vi "Stop Listener.vi"(8 "error in (no error)":errorcluster, 11 "Server Controller in":refnum<class "Server Controller.lvclass">) -> (0 "error out":errorcluster, 3 "Server Controller out":refnum<class "Server Controller.lvclass">)   [LabVIEW 2026, in "Server Controller.lvlib" / "Server Controller.lvclass"]
uses:
  Server Controller.lvclass
  <vilib>/ActorFramework/Message Enqueuer/Message Enqueuer.lvclass
  Server Controller.lvclass/Server Controller.ctl
  <vilib>/ActorFramework/Message Enqueuer/Message Enqueuer.lvclass/Message Enqueuer.ctl
  <vilib>/ActorFramework/Message Enqueuer/Enqueue.vi
  <vilib>/ActorFramework/Stop Msg/Stop Msg.lvclass
  C:/Program Files/National Instruments/LabVIEW 2026/vi.lib/ActorFramework/Message/Message.lvclass
  <vilib>/ActorFramework/Message Priority Queue/Priority Enqueue.vi
  recovery/packages/ni_lib_linked_network_actor-1.2.0.19-9492AF5A82/File Group 0/vi.lib/NI/Actors/Linked Network Actor/Linked Network Actor Messages/Disconnect Msg/Disconnect Msg.lvclass
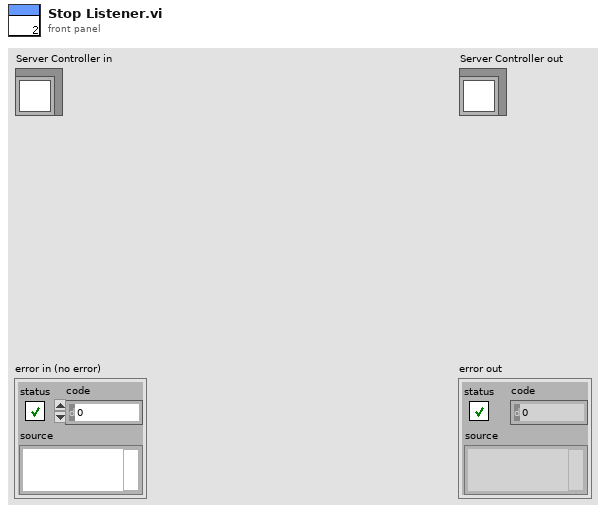
[diagram p1: front panel]
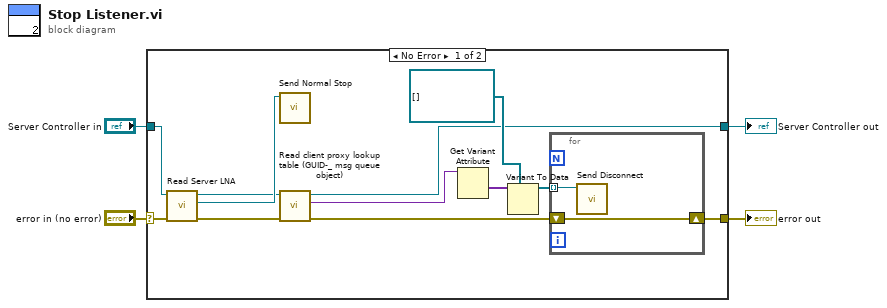
[diagram p0: block diagram]
diagram:
  n1 = case shown="No Error" "error in (no error)" {
    selector: "error in (no error)" -> [w8 w20]
    tunnel: [w5 w20] -> w3
    tunnel: [w9 w19] -> w1
    tunnel: "Server Controller in" -> [w16 w19]
    frame No Error {
      n2 = call "Read Server LNA.vi"("error in (no error)"=w8, "Server Controller in"=w16) -> ("error out"=w7:errorcluster, "Actor Framework:Message Enqueuer"=w15:refnum<class "Message Enqueuer.lvclass">, "Server Controller out"=w11:refnum<class "Server Controller.lvclass">)  [unwired: 7 in]
      n3 = call <vilib>:"Send Normal Stop.vi"("Message Enqueuer"=w15) -> ()  [unwired: 10 in, 1 out]
      n4 = call "Read client proxy lookup table (GUID-_ msg queue object).vi"("error in (no error)"=w7, "Server Controller in"=w11) -> ("error out"=w6:errorcluster, "client proxy lookup table (clientname -> msg queue object)"=w10:variant, "Server Controller out"=w9:refnum<class "Server Controller.lvclass">)  [unwired: 7 in]
      n5 = Get Variant Attribute(Variant=w10) -> (values=w12:variant[])  [unwired: 3 in, 3 out]
      n6 = Variant To Data(type=refnum<class "Message Enqueuer.lvclass">[] [], Variant=w12) -> (data=w14:refnum<class "Message Enqueuer.lvclass">[])  [unwired: 1 in, 1 out]
      n7 = for {
        tunnel: w14 -> [w18] mode=indexing
        shift-right: [w17] -> w5
        shift-left: w6 -> [w17]
        n8 = call "Send Disconnect.vi"("Message Enqueuer"=w18) -> ()  [unwired: 9 in, 2 out]
      }
    }
    frame Error {
    }
  }
  "error out" <- w3
  "Server Controller out" <- w1
